vi "Initialize Multipart Upload.vi"(8 "error in (no error)":errorcluster, 9 "PUT Object Request Parameters":T1={"Content Type"="binary/octet-stream", "ACL"=enum."private", "Storage Class"=enum."STANDARD", "User-Defined Metadata"=[]}, 10 "Object Path":string, 11 "Bucket":refnum<class "Bucket.lvclass">) -> (0 "error out":errorcluster, 3 "Multipart Upload":refnum<class "Multipart Upload.lvclass">)   [LabVIEW 2015, in "NI_AWS_S3.lvlib" / "Multipart Upload.lvclass"]
uses:
  Multipart Upload.lvclass
  Bucket/Bucket.lvclass
  PUT Object Request Parameters.ctl
  ACL.ctl
  Storage Class.ctl
  Core/HTTP Request/Name Value Pair.ctl
  Core/HTTP Request/Request Options.ctl
  Core/HTTP Request/Region handling.ctl
  Core/HTTP Request/URL formatting.ctl
  Bucket/Bucket.lvclass/Bucket.ctl
  Bucket/Read Name.vi
  Core/HTTP Request/HTTP Request.lvclass
  XML Parsing/NI_XML Parsing.lvlib
  NI_AWS_S3.lvlib
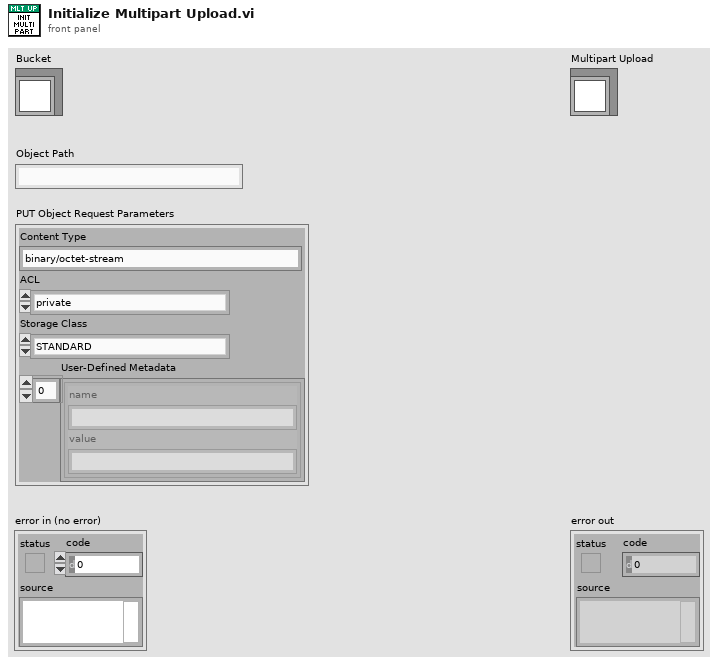
[diagram p1: front panel]
types:
  T1 = typedef "NI_AWS_S3.lvlib/PUT Object Request Parameters.ctl" = cluster{"Content Type":string, "ACL":T2, "Storage Class":T3, "User-Defined Metadata":T4[]}
  T2 = typedef "NI_AWS_S3.lvlib/ACL.ctl" = enum16{"private", "public-read", "public-read-write", "aws-exec-read", "authenticated-read", "bucket-owner-read", "bucket-owner-full-control"}
  T3 = typedef "NI_AWS_S3.lvlib/Storage Class.ctl" = enum16{"STANDARD", "REDUCED_REDUNDANCY"}
  T4 = typedef "NI_AWS_Core.lvlib/HTTP Request.lvclass/Name Value Pair.ctl" = cluster{"name":string, "value":string}
  T5 = typedef "NI_AWS_Core.lvlib/HTTP Request.lvclass/Region handling.ctl" = enum16{"use region everywhere", "use region (authentication only)", "use region (URL only)", "ignore region everwhere"}
  T6 = typedef "NI_AWS_Core.lvlib/HTTP Request.lvclass/Request Options.ctl" = cluster{"request headers":T4[], "request parameters":T4[], "request body":string, "region handling":T5, "URL formatting":T7}
  T7 = typedef "NI_AWS_Core.lvlib/HTTP Request.lvclass/URL formatting.ctl" = enum16{"region-", "region."}
  T8 = typedef "NI_AWS_Core.lvlib/HTTP Request.lvclass/Response.ctl" = cluster{"Headers":string, "Body":string}
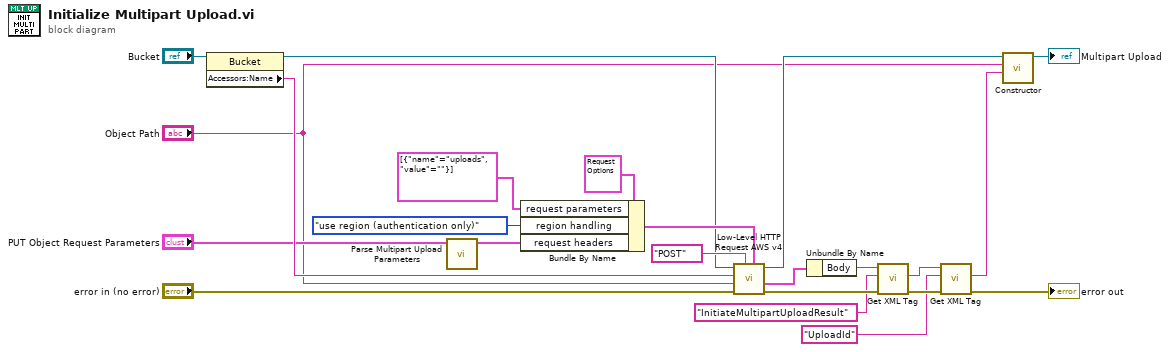
[diagram p0: block diagram]
diagram:
  n1 = property class="Bucket"(reference="Bucket") -> (reference out=w16:refnum<class "Bucket.lvclass">, "Accessors:Name"=w19:string)  [unwired: 1 in, 1 out]
  n2 = call "Parse Multipart Upload Parameters.vi"("Multipart Upload Parameters"="PUT Object Request Parameters") -> ("HTTP Headers"=w6:T4[])  [unwired: 10 in]
  n3 = Bundle By Name(cluster=T6 {"request headers"=[], "request parameters"=[], "request body"="", "region handling"=enum."use region everywhere", "URL formatting"=enum."region."} ("Request Options"), "request parameters"=T4[] [{"name"="uploads", "value"=""}] ("request headers"), "region handling"=Region_handling."use region (authentication only)", "request headers"=w6) -> (w18:T6)
  n4 = call "Low-Level HTTP Request AWS v4.vi"("Request Options"=w18, "HTTP-Verb"="POST", "error in (no error)"="error in (no error)", "URL Suffix"="Object Path", "URL Prefix"=w19, "AWS Core in"=w16) -> ("error out"=w22:errorcluster, "Response"=w13:T8, "AWS Core out"=w4:refnum<class "Bucket.lvclass">)  [unwired: 2 in, 1 out]
  n5 = Unbundle By Name(w13) -> ("Body"=w12:string)
  n6 = call "Get XML Tag.vi"("error in (no error)"=w22, "Tag name"="InitiateMultipartUploadResult", "XML String in"=w12) -> ("error out"=w14:errorcluster, "Tag value"=w9:string)  [unwired: 4 in, 3 out]
  n7 = call "Get XML Tag.vi"("error in (no error)"=w14, "Tag name"="UploadId", "XML String in"=w9) -> ("error out"=→"error out":errorcluster, "Tag value"=w1:string)  [unwired: 4 in, 3 out]
  n8 = call "Constructor.vi"("Upload ID"=w1, "Object Key"="Object Path", "Bucket"=w4) -> ("Multipart Upload"=→"Multipart Upload":refnum<class "Multipart Upload.lvclass">)  [unwired: 8 in]
